vi "NIIE_LayerCluster_ValueChange.vi"(7 "Old Visibility?":bool, 8 "Error":errorcluster, 9 "Old Name":string, 10 "CtlRef":refnum<vi>, 11 "Data":T1={"Class"={"Ants"=refnum, "Layer"=refnum, "Templates"=refnum, "Icon"=refnum, "Glyph"=refnum, "Settings"=refnum, "Tools"=refnum}, "Ref"={"Add Layer"=refnum, "Remove Layer"=refnum, "Line Text"=[], "Body Text Spec"=refnum, "DNL_Font"=refnum, "glyph path str"=refnum, "templates path str"=refnum, "Arrow Up"=refnum, "Arrow Down"=refnum, "IE VI Ref"=refnum, "Glyphs tree"=refnum, "Templates tree"=refnum, "Layer Icon Text"=refnum, "Layer Template"=refnum, "Clipboard"=refnum, "BW icon in"=refnum, "Color icon in"=refnum, "Layer Clust"=refnum, "Body Text"=refnum, "DNL_Framework Templates"=refnum, "Search Templates"=refnum, "TextMarker"=refnum, "Tab Control"=refnum, "Search Glyphs"=refnum, "Line Color"=refnum, "DNL_Glyphs []"=refnum, "Fill Color"=refnum, "Tools"=refnum, "Glyphs tree"=refnum, "Icon"=refnum, "Preview"=refnum, "Ants"=refnum, "Terminals"=refnum, "menu reference"=refnum, "LayerNames"=[], "GlyphLoadAnimation"=refnum, "TemplateLoadAnimation"=refnum, "refreshGlyphs"=refnum, "refreshTemplates"=refnum}, "Support"={"AntsRect"={"left"=0, "top"=0, "right"=0, "bottom"=0}, "Mouse Move Coords"={"Horizontal"=0, "Vertical"=0}, "Mouse Down Coords"={"Horizontal"=0, "Vertical"=0}, "Temp Coord"={"Horizontal"=0, "Vertical"=0}, "Action"=enum."Default", "Edge Color"=4914962, "Fill Color"=16860, "Mouse Down?"=FALSE, "Draft Mode?"=FALSE, "Temp Icon"=bytes[3102], "CTRL Pressed"=FALSE, "Move Selection?"=FALSE, "AntsRect Orig"={"left"=0, "top"=0, "right"=0, "bottom"=0}, "Text"="", "TM Set?"=FALSE, "Mouse inside icon?"=FALSE, "Tool (old value)"=0, "Pencil Move Color"=0, "Swap Colors?"=FALSE, "Shift pressed?"=FALSE}}) -> (0 "Error Out":errorcluster, 3 "Data Out":T1={"Class"={"Ants"=refnum, "Layer"=refnum, "Templates"=refnum, "Icon"=refnum, "Glyph"=refnum, "Settings"=refnum, "Tools"=refnum}, "Ref"={"Add Layer"=refnum, "Remove Layer"=refnum, "Line Text"=[], "Body Text Spec"=refnum, "DNL_Font"=refnum, "glyph path str"=refnum, "templates path str"=refnum, "Arrow Up"=refnum, "Arrow Down"=refnum, "IE VI Ref"=refnum, "Glyphs tree"=refnum, "Templates tree"=refnum, "Layer Icon Text"=refnum, "Layer Template"=refnum, "Clipboard"=refnum, "BW icon in"=refnum, "Color icon in"=refnum, "Layer Clust"=refnum, "Body Text"=refnum, "DNL_Framework Templates"=refnum, "Search Templates"=refnum, "TextMarker"=refnum, "Tab Control"=refnum, "Search Glyphs"=refnum, "Line Color"=refnum, "DNL_Glyphs []"=refnum, "Fill Color"=refnum, "Tools"=refnum, "Glyphs tree"=refnum, "Icon"=refnum, "Preview"=refnum, "Ants"=refnum, "Terminals"=refnum, "menu reference"=refnum, "LayerNames"=[], "GlyphLoadAnimation"=refnum, "TemplateLoadAnimation"=refnum, "refreshGlyphs"=refnum, "refreshTemplates"=refnum}, "Support"={"AntsRect"={"left"=0, "top"=0, "right"=0, "bottom"=0}, "Mouse Move Coords"={"Horizontal"=0, "Vertical"=0}, "Mouse Down Coords"={"Horizontal"=0, "Vertical"=0}, "Temp Coord"={"Horizontal"=0, "Vertical"=0}, "Action"=enum."Default", "Edge Color"=4914962, "Fill Color"=16860, "Mouse Down?"=FALSE, "Draft Mode?"=FALSE, "Temp Icon"=bytes[3102], "CTRL Pressed"=FALSE, "Move Selection?"=FALSE, "AntsRect Orig"={"left"=0, "top"=0, "right"=0, "bottom"=0}, "Text"="", "TM Set?"=FALSE, "Mouse inside icon?"=FALSE, "Tool (old value)"=0, "Pencil Move Color"=0, "Swap Colors?"=FALSE, "Shift pressed?"=FALSE}})   [LabVIEW 2021]
uses:
  MB CORE/TypeDefs/Cluster_Layer Data.ctl
  Controls/IE Data.ctl
  Class/Ants/Ants.lvclass
  Class/FakedArray/FakedArray.lvclass
  Class/Icon Library/Glyph.lvclass
  Class/Settings/Settings.lvclass
  Class/Tools/Tools Paint.lvclass
  vi.lib/LabVIEW Icon API/lv_icon/Classes/Icon/Icon.lvclass
  Controls/IE Classes.ctl
  Controls/References Cluster.ctl
  Controls/SupportClass.ctl
  <vilib>/Utility/miscctls.llb/LVPoint32TypeDef.ctl
  Controls/ENUM_SupportClass_Action.ctl
  vi.lib/LabVIEW Icon API/lv_icon/Controls/IEColor.ctl
  vi.lib/LabVIEW Icon API/lv_icon/Classes/Layer/Layer.lvclass
panel:
  in  "?":T8={"LayerIcon"=bytes[3102], "LayerName"="", "Opacity"=100, "Visibility?"=TRUE} {"Opacity" scale=0.0..100.0}
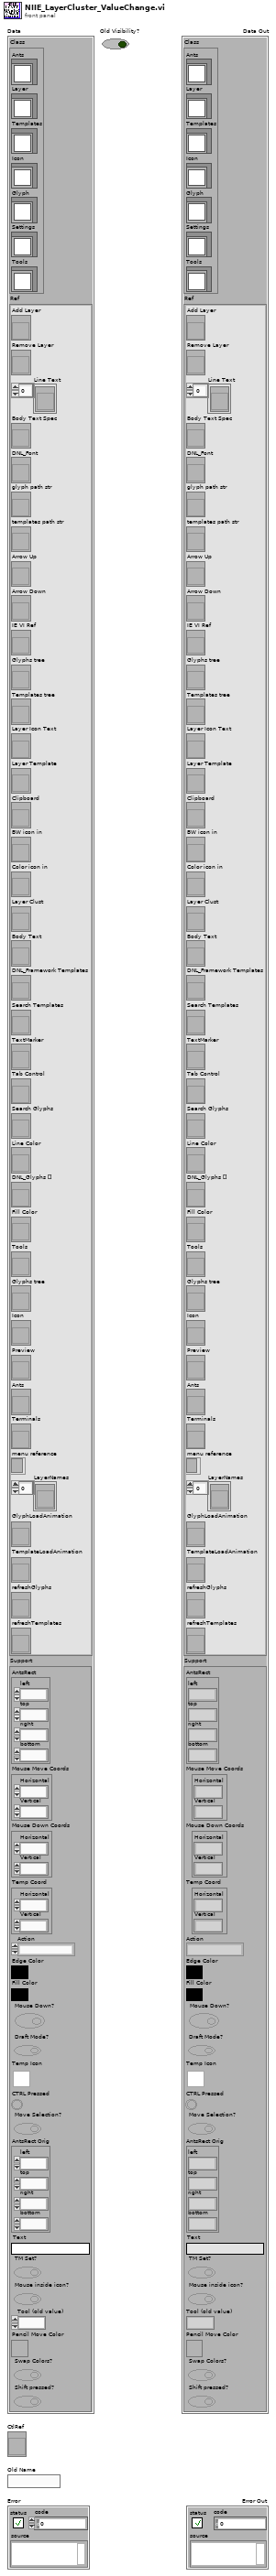
[diagram p1: front panel]
types:
  T1 = typedef "IE Data.ctl" = cluster{"Class":T2, "Ref":T3, "Support":T4}
  T2 = typedef "IE Classes.ctl" = cluster{"Ants":refnum<class "Ants.lvclass">, "Layer":refnum<class "FakedArray.lvclass">, "Templates":refnum<class "FakedArray.lvclass">, "Icon":refnum<class "Icon.lvclass">, "Glyph":refnum<class "Glyph.lvclass">, "Settings":refnum<class "Settings.lvclass">, "Tools":refnum<class "Tools Paint.lvclass">}
  T3 = typedef "References Cluster.ctl" = cluster{"Add Layer":refnum<vi>, "Remove Layer":refnum<vi>, "Line Text":refnum<vi>[], "Body Text Spec":refnum<vi>, "DNL_Font":refnum<vi>, "glyph path str":refnum<vi>, "templates path str":refnum<vi>, "Arrow Up":refnum<vi>, "Arrow Down":refnum<vi>, "IE VI Ref":refnum<vi>, "Glyphs tree":refnum<vi>, "Templates tree":refnum<vi>, "Layer Icon Text":refnum<vi>, "Layer Template":refnum<vi>, "Clipboard":refnum<vi>, "BW icon in":refnum<vi>, "Color icon in":refnum<vi>, "Layer Clust":refnum<vi>, "Body Text":refnum<vi>, "DNL_Framework Templates":refnum<vi>, "Search Templates":refnum<vi>, "TextMarker":refnum<vi>, "Tab Control":refnum<vi>, "Search Glyphs":refnum<vi>, "Line Color":refnum<vi>, "DNL_Glyphs []":refnum<vi>, "Fill Color":refnum<vi>, "Tools":refnum<vi>, "Glyphs tree":refnum<vi>, "Icon":refnum<vi>, "Preview":refnum<vi>, "Ants":refnum<vi>, "Terminals":refnum<vi>, "menu reference":refnum<k9>, "LayerNames":refnum<vi>[], "GlyphLoadAnimation":refnum<vi>, "TemplateLoadAnimation":refnum<vi>, "refreshGlyphs":refnum<vi>, "refreshTemplates":refnum<vi>}
  T4 = typedef "SupportClass.ctl" = cluster{"AntsRect":cluster{"left":i16, "top":i16, "right":i16, "bottom":i16}, "Mouse Move Coords":T5, "Mouse Down Coords":T5, "Temp Coord":T5, "Action":T6, "Edge Color":T7, "Fill Color":T7, "Mouse Down?":bool, "Draft Mode?":bool, "Temp Icon":picture, "CTRL Pressed":bool, "Move Selection?":bool, "AntsRect Orig":cluster{"left":i16, "top":i16, "right":i16, "bottom":i16}, "Text":string, "TM Set?":bool, "Mouse inside icon?":bool, "Tool (old value)":u32, "Pencil Move Color":u32, "Swap Colors?":bool, "Shift pressed?":bool}
  T5 = typedef "LVPoint32TypeDef.ctl" = cluster{"Horizontal":i32, "Vertical":i32}
  T6 = typedef "ENUM_SupportClass_Action.ctl" = enum16{"Default", "Move Selection", "Glyph Library", "Tool"}
  T7 = typedef "IEColor.ctl" = u32
  T8 = typedef "Cluster_Layer Data.ctl" = cluster{"LayerIcon":picture, "LayerName":string, "Opacity":u8, "Visibility?":bool}
  T9 = typedef "Font.ctl" = string
  T10 = typedef "Alignment.ctl" = u16
  T11 = typedef "Font Size.ctl" = u8
  T12 = cluster{"Line 1 text":string, "Line 2 text":string, "Line 3 text":string, "Line 4 text":string, "Line 1 color":u32, "Line 2 color":u32, "Line 3 color":u32, "Line 4 color":u32, "Body Text Spec":cluster{"DNL_Font":T9, "Alignment":T10, "Size":T11}, "Center text vertically":bool, "Capitalize Text":bool}
  T13 = cluster{"Horizontal":i32, "Vertical":i32, "Vertical 2":i32, "Vertical 3":i32}
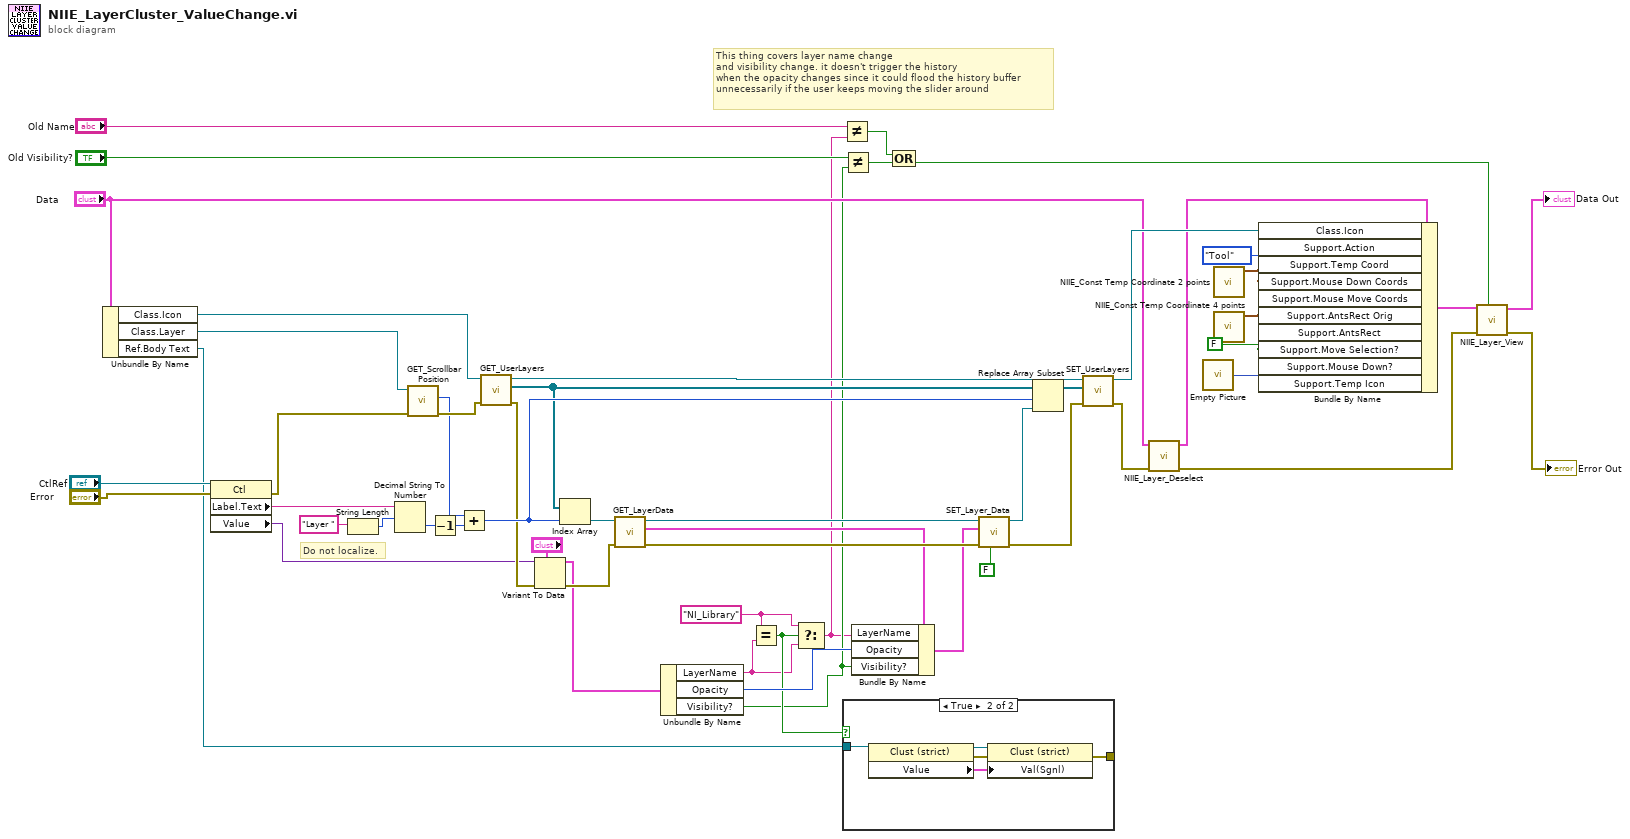
[diagram p0: block diagram]
diagram:
  w13 = "NI_Library" ("x")
  w33 = FALSE ("Mouse Down?")
  # "This thing covers layer name change\nand visibility change. it doesn't trigger the history\nwhen the opacity changes since it could flood the history buffer\nunnecessarily if the user keeps moving the slider around"
  # "Do not localize."
  n1 = Unbundle By Name("Data") -> ("Class.Icon"=w39:refnum<class "Icon.lvclass">, "Class.Layer"=w38:refnum<class "FakedArray.lvclass">, "Ref.Body Text"=w9:refnum<vi>)
  n2 = property class="Ctl"(reference="CtlRef", error in="Error") -> (error out=w29:errorcluster, "Label.Text"=w44:string, "Value"=w48:variant)  [unwired: 1 out]
  n3 = String Length(string="Layer ") -> (length=w40:i32)
  n4 = Decimal String To Number(string=w44, offset=w40) -> (number=w46:i32)  [unwired: 2 out]
  n5 = call-dynamic "GET_Scrollbar Position.vi"("error in (no error)"=w29, "FakedArray.lvclass in"=w38) -> ("error out"=w49:errorcluster, "Scrollbar Position"=w47:i32)  [unwired: 8 out]
  n6 = Decrement(x=w46) -> (x-1=w45:i32)
  n7 = Add(x=w47, y=w45) -> (x+y=w54:i32)
  n8 = call-dynamic "GET_UserLayers.vi"("error in (no error)"=w49, "Icon.lvclass in"=w39) -> ("error out"=w51:errorcluster, "All Layers"=w53:refnum<class "Layer.lvclass">[], "Icon.lvclass out"=w50:refnum<class "Icon.lvclass">)  [unwired: 7 out]
  n9 = Variant To Data(error in=w51, type="?", Variant=w48) -> (data=w12:T8, error out=w21:errorcluster)
  n10 = Index Array(array=w53, index=w54) -> (element=w23:refnum<class "Layer.lvclass">)
  n11 = call-dynamic "GET_LayerData.vi"("error in (no error)"=w21, "Layer.lvclass in"=w23) -> ("error out"=w20:errorcluster, "Data"=w14:T8, "Layer.lvclass out"=w22:refnum<class "Layer.lvclass">)  [unwired: 7 out]
  n12 = Unbundle By Name(w12) -> ("LayerName"=w8:string, "Opacity"=w11:u8, "Visibility?"=w6:bool)
  n13 = Equal?(x=w13, y=w8) -> (x = y?=w10:bool)
  n14 = Select(t=w13, s=w10, f=w8) -> (s? t:f=w4:string)
  n15 = Not Equal?(x="Old Name", y=w4) -> (x != y?=w2:bool)
  n16 = Not Equal?(x="Old Visibility?", y=w6) -> (x != y?=w5:bool)
  n17 = case shown="True" w10 {
    tunnel: w9 -> [_ w59]
    tunnel: [_ w56] -> _
    frame False {
    }
    frame True {
      n18 = property class="Clust (strict)"(reference=w59) -> (reference out=w58:refnum<vi>, error out=w55:errorcluster, "Value"=w57:T12)  [unwired: 1 in]
      n19 = property class="Clust (strict)"(reference=w58, error in=w55, "Val(Sgnl)"=w57) -> (error out=w56:errorcluster)  [unwired: 1 out]
    }
  }
  n20 = Bundle By Name(cluster=w14, "LayerName"=w4, "Opacity"=w11, "Visibility?"=w6) -> (w15:T8)
  n21 = Compound Arithmetic op=OR(w2, w5) -> (w1:bool)
  n22 = call-dynamic "SET_Layer_Data.vi"("Layer Tab Value Change? (F)"=FALSE, "error in (no error)"=w20, "Data"=w15, "Layer.lvclass in"=w22) -> ("error out"=w19:errorcluster, "Layer.lvclass out"=w18:refnum<class "Layer.lvclass">)  [unwired: 6 out]
  n23 = Replace Array Subset(array=w53, new element=w18, index=w54) -> (w16:refnum<class "Layer.lvclass">[])
  n24 = call-dynamic "SET_UserLayers.vi"("error in (no error)"=w19, "Layers"=w16, "Icon.lvclass in"=w50) -> ("error out"=w28:errorcluster, "Icon.lvclass out"=w37:refnum<class "Icon.lvclass">)  [unwired: 7 in]
  n25 = call "NIIE_Layer_Deselect.vi"("Error"=w28, "Data"="Data") -> ("Error Out"=w25:errorcluster, "Data Out"=w30:T1)  [unwired: 8 out]
  n26 = call "Empty Picture"() -> ("empty picture"=w32:picture)
  n27 = call "NIIE_Const Temp Coordinate 2 points.vi"() -> ("Const Temp Coordinate"=w35:T5)  [unwired: 11 out]
  n28 = call "NIIE_Const Temp Coordinate 4 points.vi"() -> ("Const Temp Coordinate"=w34:T13)  [unwired: 11 out]
  n29 = Bundle By Name(cluster=w30, "Class.Icon"=w37, "Support.Action"=ENUM_SupportClass_Action."Tool" ("Action"), "Support.Temp Coord"=w35, "Support.Mouse Down Coords"=w35, "Support.Mouse Move Coords"=w35, "Support.AntsRect Orig"=w34, "Support.AntsRect"=w34, "Support.Move Selection?"=w33, "Support.Mouse Down?"=w33, "Support.Temp Icon"=w32) -> (w27:T1)
  n30 = call "NIIE_Layer_View.vi"("Add To Undo?"=w1, "Error"=w25, "Data"=w27) -> ("Error Out"=→"Error Out":errorcluster, "Data Out"=→"Data Out":T1)  [unwired: 2 in, 5 out]
